vi "stitchingModeAverage.vi"(9 "Data In":dbl[][][](array[numeric])) -> (2 "Data Out":dbl[][](array[numeric]))   [LabVIEW 2020, in "horiba.lvlib" / "CCD.lvclass"]
doc: "Stitches spectra based on simple cut-off modus."
uses:
  CCD.lvclass
  9502b2a2-e153-4c02-8d5e-41dccb573229.vi
  <vilib>/Array/Sort 2D Array - Pop Stack.vi
  <vilib>/Array/Sort 2D Array - Push Stack.vi
  9502b2a2-e153-4c02-8d5e-41dccb573229.vi/269d4b3b-47f5-49e3-8884-44851e4dd9d5.vi
  9502b2a2-e153-4c02-8d5e-41dccb573229.vi/6d99389c-673d-4efb-bf33-19b32bcf4cf8.vi
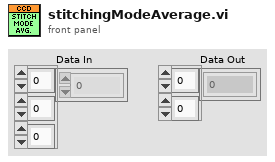
[diagram p1: front panel]
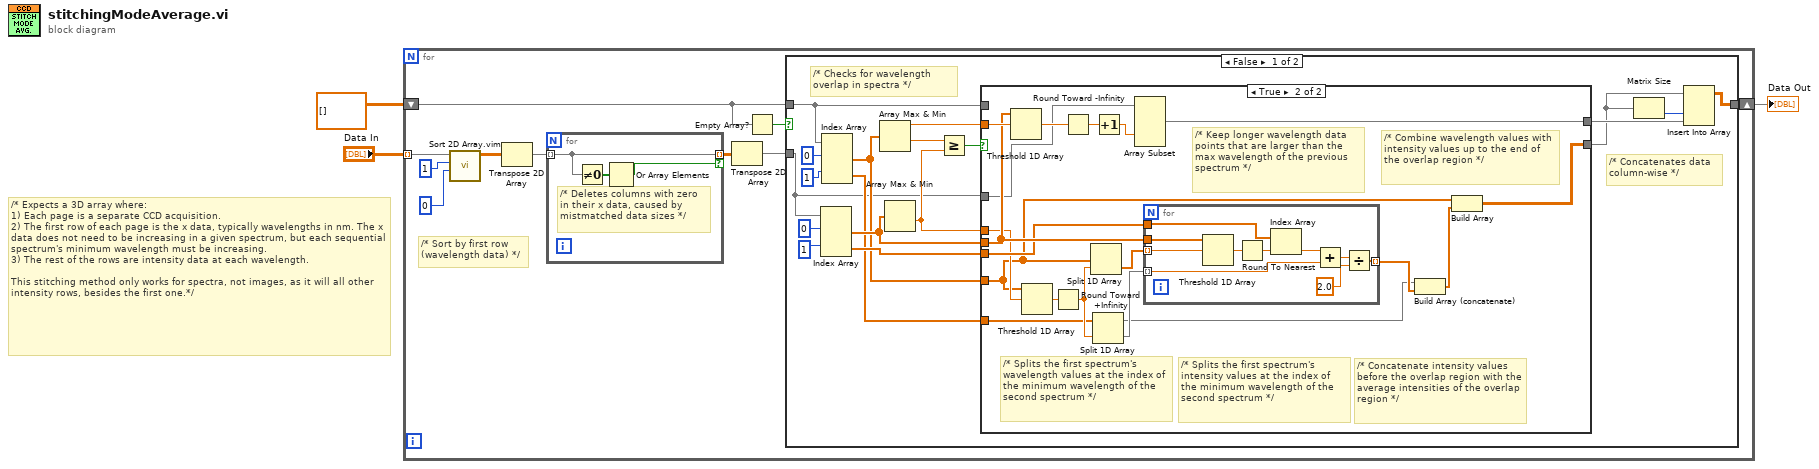
[diagram p0: block diagram]
diagram:
  # "/* Expects a 3D array where:\n1) Each page is a separate CCD acquisition.\n2) The first row of each page is the x data, typically wavelengths in nm. The x data does not need to be increasing in a given spectrum, but each sequential spectrum's minimum wavelength must be increasing.\n3) The rest of the rows are intensity data at each wavelength. \n\nThis stitching method only works for spectra, not images, as it will all other intensity rows, besides the first one.*/"
  n1 = for {
    tunnel: "Data In" -> [w7] mode=indexing
    shift-right: [w13] -> w3
    shift-left: dbl[][] [] ("Empty Array") -> [w4]
    # "/* Sort by first row \n(wavelength data) */"
    n2 = call "Sort 2D Array.vim"("index"=0, "dimension to index (column)"=1 ("index"), "2D array"=w7) -> ("sorted 2D array"=w5:dbl[][])  [unwired: 7 in, 1 out]
    n3 = Transpose 2D Array(2D array=w5) -> (transposed array=w11:dbl[][])
    n4 = for {
      tunnel: w11 -> [w15] mode=indexing
      tunnel: [w15] -> w10 mode=indexing if=w16
      # "/* Deletes columns with zero\nin their x data, caused by\nmistmatched data sizes */"
      n5 = Not Equal To 0?(x=w15) -> (x != 0?=w14:bool[])
      n6 = Or Array Elements(Boolean array=w14) -> (logical OR=w16:bool)
    }
    n7 = Transpose 2D Array(2D array=w10) -> (transposed array=w6:dbl[][])
    n8 = Empty Array?(array=w4) -> (empty?=w12:bool)
    n9 = case shown="False" w12 {
      tunnel: [w27 w65] -> w13
      tunnel: w6 -> [w18 w65]
      tunnel: w4 -> [w20 _]
      frame False {
        # "/* Concatenates data \ncolumn-wise */"
        # "/* Checks for wavelength \noverlap in spectra */"
        n10 = Index Array(array=w18, index (row) #1=0 ("index (row)"), index (row) #2=1 ("index (row)")) -> (element #1=w24:dbl[], element #2=w23:dbl[])  [unwired: 2 in]
        n11 = Index Array(array=w20, index (row) #1=0 ("index (row)"), index (row) #2=1 ("index (row)")) -> (element #1=w21:dbl[], element #2=w19:dbl[])  [unwired: 2 in]
        n12 = Array Max & Min(array=w21) -> (max value=w29:dbl)  [unwired: 3 out]
        n13 = Array Max & Min(array=w24) -> (min value=w22:dbl)  [unwired: 3 out]
        n14 = Greater Or Equal?(x=w29, y=w22) -> (x >= y?=w28:bool)
        n15 = case shown="True" w28 {
          tunnel: w18 -> [w35 w37]
          tunnel: [w35 w54] -> w30
          tunnel: w24 -> [_ w49]
          tunnel: w29 -> [_ w53]
          tunnel: w23 -> [_ w48]
          tunnel: w22 -> [_ w47]
          tunnel: w21 -> [_ w39]
          tunnel: w20 -> [w34 _]
          tunnel: [w34 w36] -> w17
          tunnel: w19 -> [_ w38]
          frame False {
            # "/* Passes new data unmodified if \nthere is no overlap */"
          }
          frame True {
            # "/* Splits the first spectrum's intensity values at the index of the minimum wavelength of the second spectrum */"
            # "/* Combine wavelength values with intensity values up to the end of the overlap region */"
            # "/* Concatenate intensity values before the overlap region with the average intensities of the overlap region */"
            # "/* Splits the first spectrum's wavelength values at the index of the minimum wavelength of the second spectrum */"
            # "/* Keep longer wavelength data points that are larger than the max wavelength of the previous spectrum */"
            n16 = Threshold 1D Array(2:w53, 3:w49) -> (0:w51:dbl)  [unwired: 1 in]
            n17 = Threshold 1D Array(2:w47, 3:w39) -> (0:w46:dbl)  [unwired: 1 in]
            n18 = Round Toward +Infinity(x=w46) -> (ceil(x): smallest int >= x=w44:dbl)
            n19 = Round Toward -Infinity(1:w51) -> (0:w52:dbl)
            n20 = Split 1D Array(array=w39, index=w44) -> (second subarray=w45:dbl[])  [unwired: 1 out]
            n21 = Split 1D Array(array=w38, index=w44) -> (first subarray=w41:dbl[], second subarray=w43:dbl[])
            n22 = Increment(x=w52) -> (x+1=w50:dbl)
            n23 = Array Subset(array=w37, index (col)=w50) -> (w54:dbl[][])  [unwired: 3 in]
            n24 = for {
              tunnel: w49 -> [w62]
              tunnel: w48 -> [w61]
              tunnel: w45 -> [w60] mode=indexing
              tunnel: w43 -> [w59] mode=indexing
              tunnel: [w55] -> w42 mode=indexing
              n25 = Threshold 1D Array(2:w60, 3:w62) -> (0:w64:dbl)  [unwired: 1 in]
              n26 = Round To Nearest(number=w64) -> (nearest integer value=w63:dbl)
              n27 = Index Array(array=w61, index=w63) -> (element=w58:dbl)
              n28 = Add(x=w58, y=w59) -> (x+y=w57:dbl)
              n29 = Divide(x=w57, y=2.0) -> (x/y=w55:dbl)
            }
            n30 = Build Array (concatenate)(w41, w42) -> (w40:dbl[])
            n31 = Build Array(w39, w40) -> (w36:dbl[][])
          }
        }
        n32 = Matrix Size(0:w17) -> (2:w31:i32)  [unwired: 1 out]
        n33 = Insert Into Array(array=w17, index (col)=w31, new element=w30) -> (w27:dbl[][])  [unwired: 1 in]
      }
      frame True {
        # "/* This case will run on the first loop iteration */"
      }
    }
  }
  "Data Out" <- w3
